vi "Read ctl.vi"(8 "error in (no error)":errorcluster, 11 "TEC in":refnum<class "TEC.lvclass">) -> (0 "error out":errorcluster, 2 "ctl":cluster{"p":dbl, "i":dbl, "d":dbl}, 3 "TEC out":refnum<class "TEC.lvclass">)   [LabVIEW 2014, in "Generic TEC.lvlib" / "TEC.lvclass"]
uses:
  TEC.lvclass
  TEC.lvclass/TEC.ctl
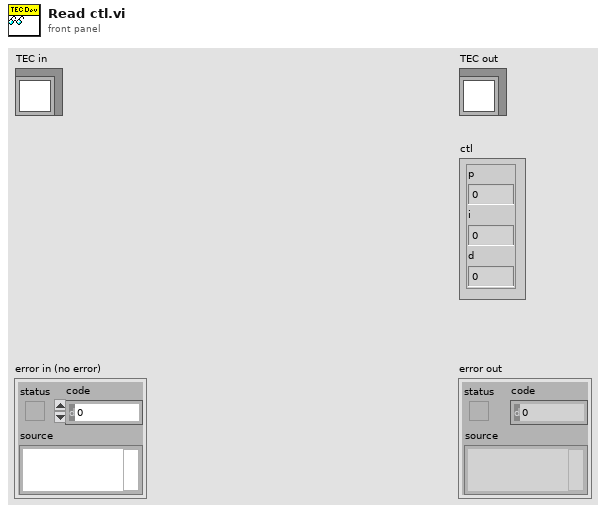
[diagram p1: front panel]
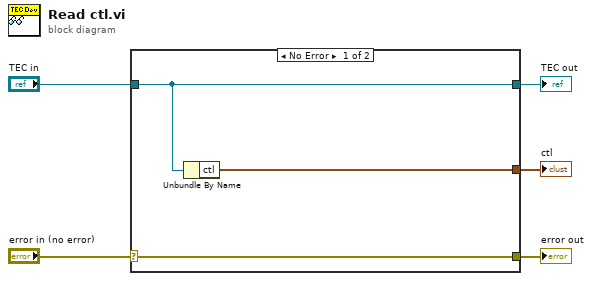
[diagram p0: block diagram]
diagram:
  n1 = case shown="No Error" "error in (no error)" {
    selector: "error in (no error)" -> [w8 w9]
    tunnel: [w8 w9] -> w4
    tunnel: [w7 w10] -> w2
    tunnel: "TEC in" -> [w7 w10]
    tunnel: [w6 _] -> w1
    frame No Error {
      n2 = Unbundle By Name(w7) -> ("ctl"=w6:cluster{"p":dbl, "i":dbl, "d":dbl})
    }
    frame Error {
    }
  }
  "error out" <- w4
  "TEC out" <- w2
  "ctl" <- w1
